vi "read-block.vi"(11 "Byte Stream File in":refnum<file>) -> (2 "Array":dbl[](array[numeric]), 3 "Byte Stream File out":refnum<file>)   [LabVIEW 2011]
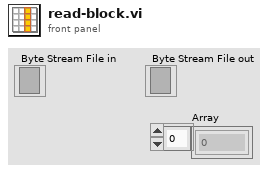
[diagram p1: front panel]
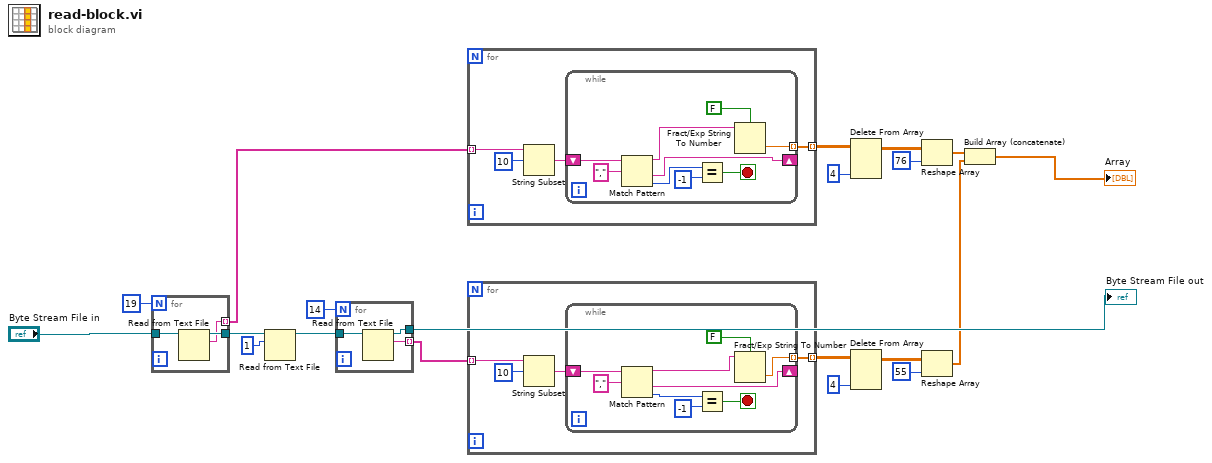
[diagram p0: block diagram]
diagram:
  n1 = for {
    N: 19 ("Numeric") -> [_]
    tunnel: "Byte Stream File in" -> [w23]
    tunnel: [w22] -> w2
    tunnel: [w21] -> w4 mode=indexing
    n2 = Read from Text File(file (use dialog)=w23) -> (refnum out=w22:refnum<file>, text=w21:string)  [unwired: 3 in, 2 out]
  }
  n3 = Read from Text File(file (use dialog)=w2, count=1) -> (refnum out=w8:refnum<file>)  [unwired: 2 in, 3 out]
  n4 = for {
    N: 14 ("Numeric") -> [_]
    tunnel: w8 -> [w26]
    tunnel: [w25] -> w20
    tunnel: [w24] -> w10 mode=indexing
    n5 = Read from Text File(file (use dialog)=w26) -> (refnum out=w25:refnum<file>, text=w24:string)  [unwired: 3 in, 2 out]
  }
  "Byte Stream File out" <- w20
  n6 = for {
    tunnel: w4 -> [w28] mode=indexing
    tunnel: [w29] -> w5 mode=indexing
    n7 = String Subset(string=w28, offset (0)=10) -> (substring=w27:string)  [unwired: 1 in]
    n8 = while {
      shift-right: [w37] -> _
      shift-left: w27 -> [w39]
      tunnel: [w36] -> w29 mode=indexing
      stop <- w33 stop-if-true
      n9 = Match Pattern(string=w39, regular expression=",") -> (before substring=w38:string, after substring=w37:string, offset past match=w35:i32)  [unwired: 1 in, 1 out]
      n10 = Equal?(x=w35, y=-1) -> (x = y?=w33:bool)
      n11 = Fract/Exp String To Number(use system decimal point (T)=FALSE, string=w38) -> (number=w36:dbl)  [unwired: 2 in, 1 out]
    }
  }
  n12 = for {
    tunnel: w10 -> [w41] mode=indexing
    tunnel: [w42] -> w11 mode=indexing
    n13 = String Subset(string=w41, offset (0)=10) -> (substring=w40:string)  [unwired: 1 in]
    n14 = while {
      shift-right: [w50] -> _
      shift-left: w40 -> [w52]
      tunnel: [w49] -> w42 mode=indexing
      stop <- w46 stop-if-true
      n15 = Match Pattern(string=w52, regular expression=",") -> (before substring=w51:string, after substring=w50:string, offset past match=w48:i32)  [unwired: 1 in, 1 out]
      n16 = Equal?(x=w48, y=-1) -> (x = y?=w46:bool)
      n17 = Fract/Exp String To Number(use system decimal point (T)=FALSE, string=w51) -> (number=w49:dbl)  [unwired: 2 in, 1 out]
    }
  }
  n18 = Delete From Array(array=w5, index (col)=4 ("disabled index (col)")) -> (array with subset deleted=w13:dbl[][])  [unwired: 2 in, 1 out]
  n19 = Delete From Array(array=w11, index (col)=4 ("disabled index (col)")) -> (array with subset deleted=w16:dbl[][])  [unwired: 2 in, 1 out]
  n20 = Reshape Array(w13, 76 ("dimension size")) -> (w17:dbl[])
  n21 = Reshape Array(w16, 55 ("dimension size")) -> (w18:dbl[])
  n22 = Build Array (concatenate)(w17, w18) -> (→"Array":dbl[])
